vi "DigitalOutputStart.vi"(0 "Device Info":T1={"Serial Number"=-1, "Channel"=0, "Port"=0}, 1 "LEDForwardVoltage":u32(ring)=2 items=["LED_FORWARD_VOLTAGE_1_7V"=1, "LED_FORWARD_VOLTAGE_2_75V"=2, "LED_FORWARD_VOLTAGE_3_2V"=3, "LED_FORWARD_VOLTAGE_3_9V"=4, "LED_FORWARD_VOLTAGE_4_0V"=5, "LED_FORWARD_VOLTAGE_4_8V"=6, "LED_FORWARD_VOLTAGE_5_0V"=7, "LED_FORWARD_VOLTAGE_5_6V"=8], 2 "Current Limit":dbl=0.02 caption="LED Current Limit", 5 "IsHubPort":bool, 11 "error in (no error)":errorcluster, 12 "Connection":u16(ring) items=["No Preference", "Remote", "Local"], 13 "Timeout (mSec)":i32=5000) -> (4 "Phidget ID":u64, 6 "Serial Number Return":i32, 10 "Attached?":bool, 15 "error out":errorcluster)   [LabVIEW 2012, in "Phidget Digital Output.lvlib"]
doc: "${DigitalOutput:StartHeader}"
uses:
  <instrlib>/Phidgets/Phidget Digital Output/Phidget Digital Output.lvlib
  <instrlib>/Phidgets/Phidget Common/Phidget Common.lvlib
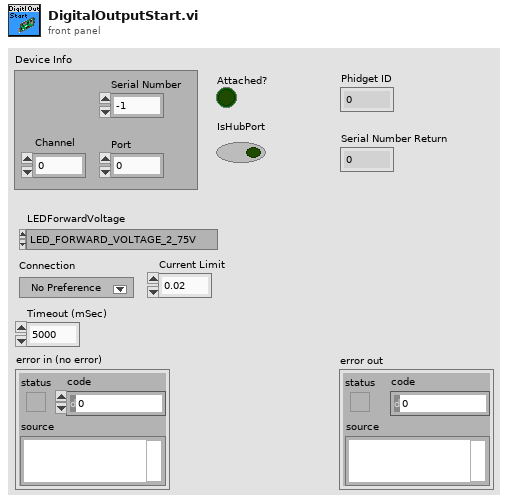
[diagram p1: front panel]
types:
  T1 = cluster{"Serial Number":i32, "Channel":i32, "Port":i32}
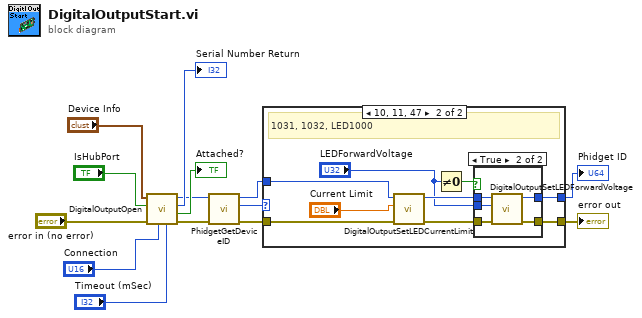
[diagram p0: block diagram]
diagram:
  n1 = call <instrlib>:"DigitalOutputOpen.vi"("Timeout (mSec)"="Timeout (mSec)", "Connection"="Connection", "error in"="error in (no error)", "IsHubPort"="IsHubPort", "Device Info"="Device Info") -> ("error out"=w5:errorcluster, "Attached?"=→"Attached?":bool, "Serial Number Return"=→"Serial Number Return":i32, "Phidget ID"=w4:u64)  [unwired: 3 in]
  n2 = call <instrlib>:"PhidgetGetDeviceID.vi"("error in (no error)"=w5, "Device In"=w4) -> ("error out"=w7:errorcluster, "Devie IDs"=w6:u32, "Device Out"=w8:u64)  [unwired: 6 in]
  n3 = case shown="10, 11, 47" w6 {
    tunnel: w7 -> [w16 w25]
    tunnel: [w16 w21] -> w2
    tunnel: w8 -> [w15 w24]
    tunnel: [w15 w20] -> w3
    frame 0, Default {
      # "Do not set device-specific\nparameters on devices that\ndon't support them"
    }
    frame 16, 17, 71 {
      # "1031, 1032, LED1000"
      n4 = call <instrlib>:"DigitalOutputSetLEDCurrentLimit.vi"("error in (no error)"=w25, "Current Limit"="Current Limit", "Device In"=w24) -> ("error out"=w22:errorcluster, "Device Out"=w23:u64)  [unwired: 6 in]
      n5 = Not Equal To 0?(x="LEDForwardVoltage") -> (x != 0?=w18:bool)
      n6 = case shown="True" w18 {
        tunnel: w23 -> [w27 w32]
        tunnel: w22 -> [w26 w31]
        tunnel: [w26 w30] -> w21
        tunnel: [w27 w29] -> w20
        tunnel: "LEDForwardVoltage" -> [_ w28]
        frame False {
        }
        frame True {
          n7 = call <instrlib>:"DigitalOutputSetLEDForwardVoltage.vi"("error in (no error)"=w31, "LEDForwardVoltage"=w28, "Device In"=w32) -> ("error out"=w30:errorcluster, "Device Out"=w29:u64)  [unwired: 6 in]
        }
      }
    }
  }
  "error out" <- w2
  "Phidget ID" <- w3
